vi "Query Voltage.vi"(8 "error in (no error)":errorcluster, 11 "Keithley 24xx in":refnum<class "Keithley 24xx.lvclass">) -> (0 "error out":errorcluster, 2 "Voltage":dbl, 3 "Keithley 24xx out":refnum<class "Keithley 24xx.lvclass">)   [LabVIEW 2020, in "Keithley 24xx.lvclass"]
uses:
  Keithley 24xx.lvclass
  C:/Sandbox/Git_Sandbox/WiSpry Test Framework source code (LV20)/WiSpry Test Framework/Instruments/Instrument.lvclass
  Instrument.lvclass/Instrument.ctl
  <instrlib>/Keithley 24XX/Public/Data/Read (Single Point).vi
  Instrument.lvclass
  <instrlib>/Keithley 24XX/Keithley 24XX.lvlib
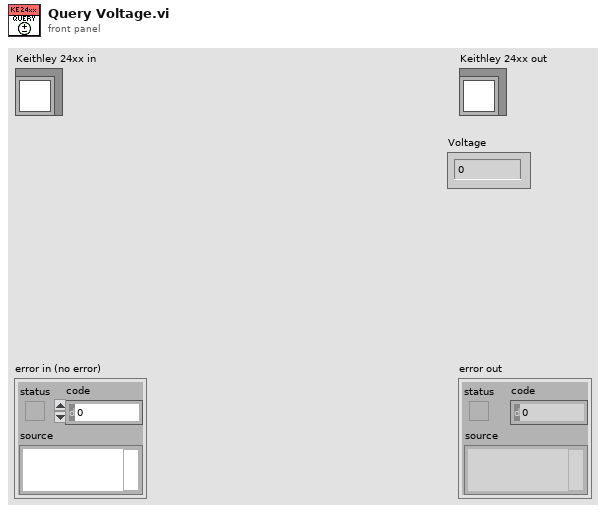
[diagram p1: front panel]
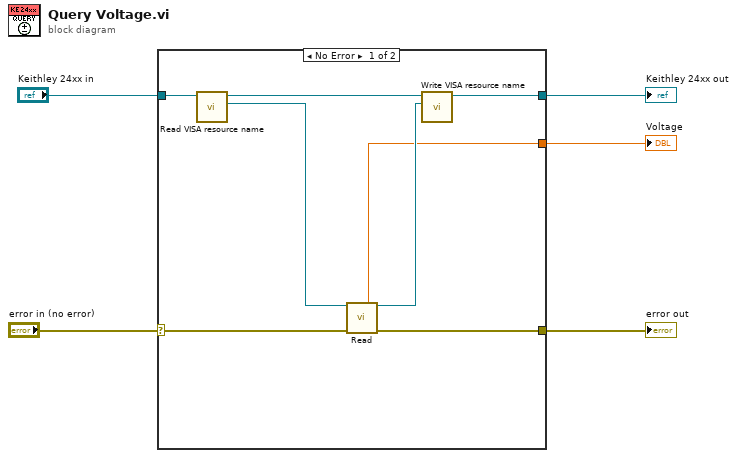
[diagram p0: block diagram]
diagram:
  n1 = case shown="No Error" "error in (no error)" {
    selector: "error in (no error)" -> [w10 w15]
    tunnel: [w7 w15] -> w1
    tunnel: [w11 w14] -> w3
    tunnel: "Keithley 24xx in" -> [w13 w14]
    tunnel: [w6 _] -> w2
    frame No Error {
      n2 = call "Read VISA resource name.vi"("Instrument in"=w13) -> ("VISA resource name"=w9:refnum<visa-resource-name>, "Instrument out"=w12:refnum<class "Keithley 24xx.lvclass">)  [unwired: 9 in]
      n3 = call-poly <instrlib>:"Read.vi"("VISA resource name"=w9, "error in (no error)"=w10) -> ("Voltage"=w6:sgl, "VISA resource name out"=w8:refnum<visa-resource-name>, "error out"=w7:errorcluster)  [unwired: 7 in, 4 out]
      n4 = call "Write VISA resource name.vi"("VISA resource name"=w8, "Instrument in"=w12) -> ("Instrument out"=w11:refnum<class "Keithley 24xx.lvclass">)  [unwired: 9 in]
    }
    frame Error {
    }
  }
  "error out" <- w1
  "Keithley 24xx out" <- w3
  "Voltage" <- w2
